vi "Progress Window Cancel.vi"(8 "error in (no error)":errorcluster, 11 "DVRs in":T1) -> (0 "error out":errorcluster, 2 "cancelled":bool, 3 "DVRs out":T1)   [LabVIEW 2019, in "Build Automation.lvlib"]
uses:
  Build Automation.lvlib
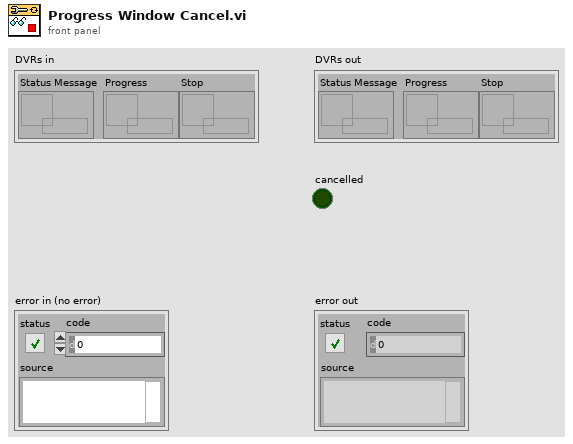
[diagram p1: front panel]
types:
  T1 = cluster{"Status Message":refnum<data-value>, "Progress":refnum<data-value>, "Stop":refnum<data-value>}
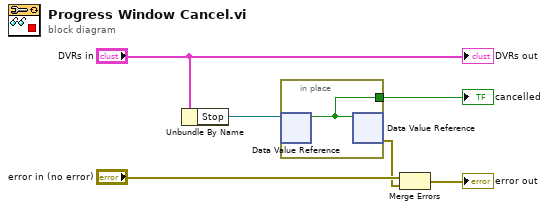
[diagram p0: block diagram]
diagram:
  n1 = Unbundle By Name("DVRs in") -> ("Stop"=w6:refnum<data-value>)
  n2 = in-place {
    in-place-border: [w7] -> w1
    n3 = in-place-dvr #1(w6) -> (w7:bool)  [unwired: 1 out]
    n4 = in-place-dvr #1(w7) -> (w4:errorcluster)  [unwired: 1 out]
  }
  "cancelled" <- w1
  n5 = Merge Errors("error in (no error)", w4) -> (→"error out":errorcluster)
  "DVRs out" <- "DVRs in"
